vi "mupEvalBulk.vi"(8 "error in (no error)":errorcluster, 10 "a_res":dbl[](array[numeric]), 11 "hParser in":u64) -> (0 "error out":errorcluster, 2 "results":dbl[](array[numeric]), 3 "hParser out":u64)   [LabVIEW 2018, in "mupLib.lvlib"]
doc: "Evaluate the expression in bult mode. Returns the array of results.\n\nIf multiple expressions have been input, the last expression will be evaluated."
uses:
  mupLib.lvlib
  <vilib>/Utility/error.llb/Error Cluster From Error Code.vi
  libmuparser-lv.dll
panel:
  # "Evaluate the expression in bult mode. Returns the array of results.\n\nIf multiple expressions have been input, the last expression will be evaluated."
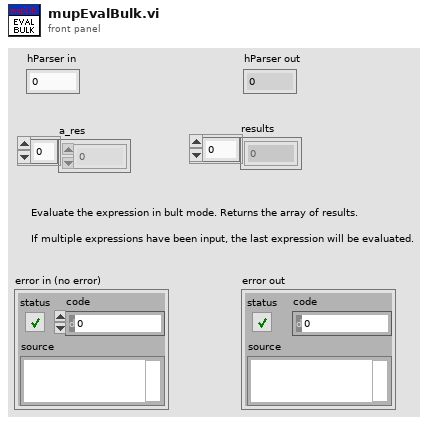
[diagram p1: front panel]
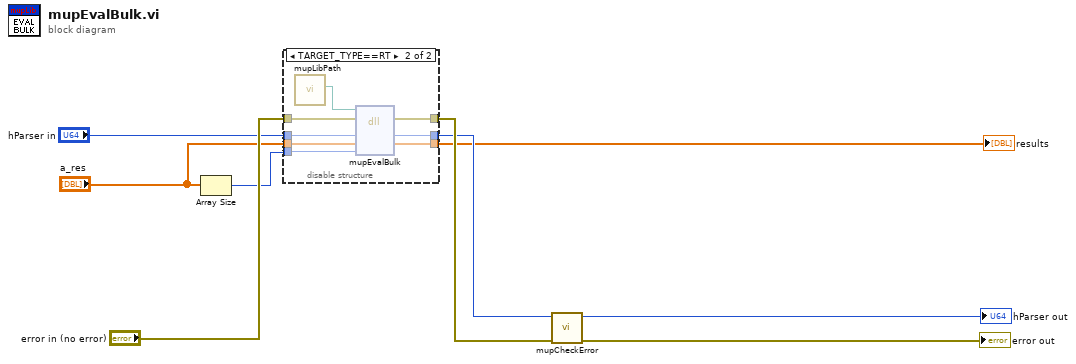
[diagram p0: block diagram]
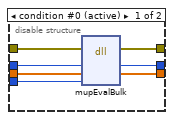
[diagram p2: hidden frame]
diagram:
  n1 = Array Size(array="a_res") -> (size(s)=w3:i32)
  n2 = disable-structure shown="TARGET_TYPE==RT" {
    disable-tunnel: [w16 w24] -> w9
    disable-tunnel: "error in (no error)" -> [w15 w23]
    disable-tunnel: "hParser in" -> [w14 w22]
    disable-tunnel: [w13 w21] -> w5
    disable-tunnel: "a_res" -> [w12 w20]
    disable-tunnel: w3 -> [w11 w19]
    disable-tunnel: [w10 w18] -> w1
    frame condition #0 (active) {
      n3 = dll-call lib="C:/Users/leonidas/Documents/GitHub/LV-muParser/mupLib/libmuparser-lv.dll" fn="mupEvalBulk"(error in=w15, "hParser"=w14, "a_res"=w12, "nSize"=w11) -> (error out=w16:errorcluster, "hParser"=w13:u64, "a_res"=w10:dbl[])  [unwired: 4 in, 1 out]
    }
    frame condition #1 {
      n4 = call "mupLibPath.vi"() -> ("libmuparser path"=w17:path)  [unwired: 11 in]
      n5 = dll-call lib="C:/Users/leonidas/Documents/GitHub/LV-muParser/mupLib/libmuparser-lv.dll" fn="mupEvalBulk"(path in=w17, error in=w23, "hParser"=w22, "a_res"=w20, "nSize"=w19) -> (error out=w24:errorcluster, "hParser"=w21:u64, "a_res"=w18:dbl[])  [unwired: 3 in, 1 out]
    }
  }
  "results" <- w1
  n6 = call "mupCheckError.vi"("error in (no error)"=w9, "hParser in"=w5) -> ("error out"=→"error out":errorcluster, "hParser out"=→"hParser out":u64)  [unwired: 8 in]
